vi "lowpassFilter.vi"(8 "in_k":dbl, 10 "TS":dbl, 11 "TF":dbl) -> (3 "filter output":dbl)   [LabVIEW 2022 SP3]
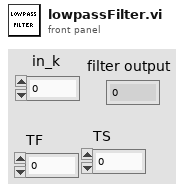
[diagram p1: front panel]
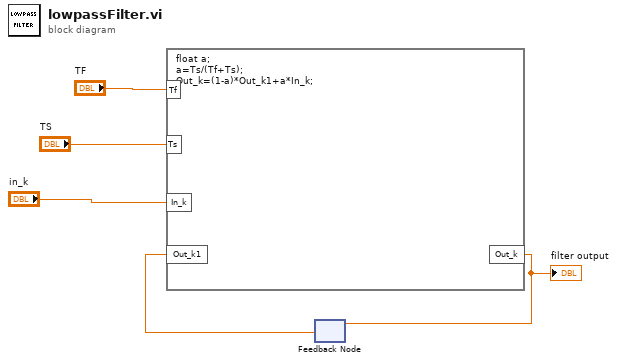
[diagram p0: block diagram]
diagram:
  n1 = feedback #1() -> (w1:dbl)  [unwired: 1 in]
  n2 = formula code="float a;\na=Ts/(Tf+Ts);\nOut_k=(1-a)*Out_k1+a*In_k;"("Tf"="TF", "Ts"="TS", "In_k"="in_k", "Out_k1"=w1) -> ("Out_k"=w2:dbl)
  "filter output" <- w2
  n3 = feedback-in #1(w2) -> ()
